vi "DC(P+V)control_KNRm.vi"(8 "control":T2, 9 "Ocmd":dbl, 10 "Tcmd":dbl, 11 "Move":T1) -> (0 "hldU":dbl, 1 "hldVerr":dbl, 2 "dirU":dbl, 3 "dirVerr":dbl, 4 "e":dbl, 5 "FriectH":dbl, 6 "dirPerr":dbl, 7 "FriectD":dbl)   [LabVIEW 2013]
uses:
  Global_KNRm.vi
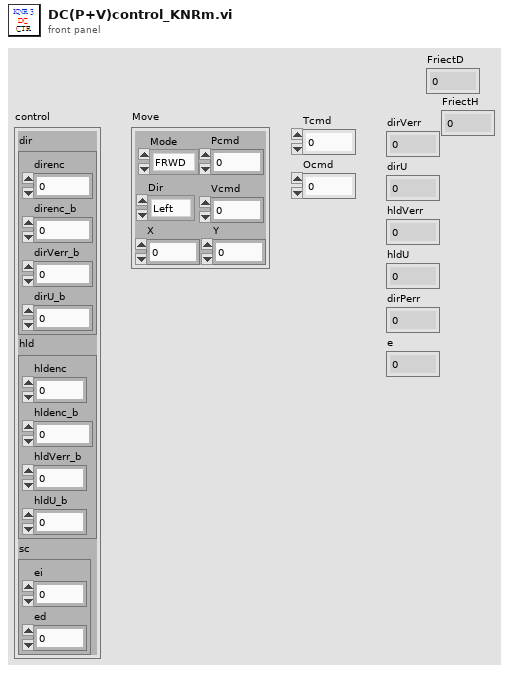
[diagram p1: front panel]
types:
  T1 = cluster{"Mode":enum16{"FRWD", "TURFIX", "TURNOF", "CIRCULAR"}, "Dir":enum16{"Left", "Right"}, "Pcmd":dbl, "Vcmd":dbl, "X":dbl, "Y":dbl}
  T2 = cluster{"dir":cluster{"direnc":dbl, "direnc_b":dbl, "dirVerr_b":dbl, "dirU_b":dbl}, "hld":cluster{"hldenc":dbl, "hldenc_b":dbl, "hldVerr_b":dbl, "hldU_b":dbl}, "sc":cluster{"ei":dbl, "ed":dbl}}
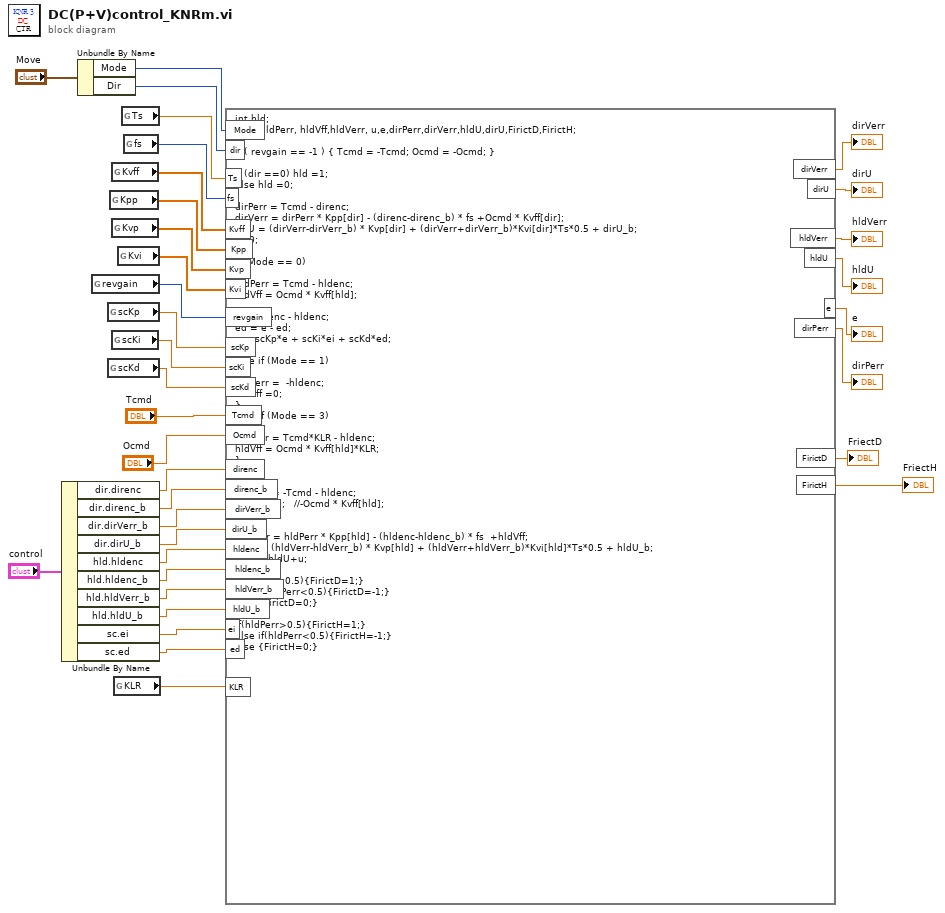
[diagram p0: block diagram]
diagram:
  n1 = Unbundle By Name("control") -> ("dir.direnc"=w19:dbl, "dir.direnc_b"=w18:dbl, "dir.dirVerr_b"=w17:dbl, "dir.dirU_b"=w16:dbl, "hld.hldenc"=w15:dbl, "hld.hldenc_b"=w14:dbl, "hld.hldVerr_b"=w13:dbl, "hld.hldU_b"=w12:dbl, "sc.ei"=w11:dbl, "sc.ed"=w10:dbl)
  n2 = Unbundle By Name("Move") -> ("Mode"=w33:enum16{"FRWD", "TURFIX", "TURNOF", "CIRCULAR"}, "Dir"=w32:enum16{"Left", "Right"})
  n3 = global read "Global_KNRm.vi" "revgain"() -> (w23:i32)
  n4 = global read "Global_KNRm.vi" "scKp"() -> (w22:dbl)
  n5 = global read "Global_KNRm.vi" "scKd"() -> (w20:dbl)
  n6 = global read "Global_KNRm.vi" "Kpp"() -> (w27:dbl[])
  n7 = global read "Global_KNRm.vi" "Kvff"() -> (w29:dbl[])
  n8 = global read "Global_KNRm.vi" "Kvp"() -> (w25:dbl[])
  n9 = global read "Global_KNRm.vi" "scKi"() -> (w21:dbl)
  n10 = global read "Global_KNRm.vi" "KLR"() -> (w1:dbl)
  n11 = global read "Global_KNRm.vi" "Kvi"() -> (w24:dbl[])
  n12 = global read "Global_KNRm.vi" "Ts"() -> (w28:dbl)
  n13 = global read "Global_KNRm.vi" "fs"() -> (w26:i32)
  n14 = formula code="int hld;\nfloat hldPerr, hldVff,hldVerr, u,e,dirPerr,dirVerr,hldU,dirU,FirictD,FirictH;\n\nif ( revgain == -1 ) { Tcmd = -Tcmd; Ocmd = -Ocmd; }\n\nif (dir ==0) hld =1;\nelse hld =0;\n\ndirPerr = Tcmd - direnc;\ndirVerr = dirPerr * Kpp[dir] - (direnc-direnc_b) * fs +Ocmd * Kvff[dir];\ndirU = (dirVerr-dirVerr_b) * Kvp[dir] + (dirVerr+dirVerr_b)*Kvi[dir]*Ts*0.5 + dirU_b;\nu=0;\n\nif (Mode == 0)\n{\nhldPerr = Tcmd - hldenc;\nhldVff = Ocmd * Kvff[hld];\n\ne = direnc - hldenc;\ned = e - ed;\nu = scKp*e + scKi*ei + scKd*ed;\n}\nelse if (Mode == 1)\n{\nhldPerr =  -hldenc;\nhldVff =0;\n}\nelse if (Mode == 3)\n{\nhldPerr = Tcmd*KLR - hldenc;\nhldVff = Ocmd * Kvff[hld]*KLR;\n}\nelse\n{\nhldPerr = -Tcmd - hldenc;\nhldVff = 0;   //-Ocmd * Kvff[hld];\n}\n\nhldVerr = hldPerr * Kpp[hld] - (hldenc-hldenc_b) * fs  +hldVff;\nhldU = (hldVerr-hldVerr_b) * Kvp[hld] + (hldVerr+hldVerr_b)*Kvi[hld]*Ts*0.5 + hldU_b;\nhldU =hldU+u;\n\nif(dirPerr>0.5){FirictD=1;}\nelse if(dirPerr<0.5){FirictD=-1;}\nelse {FirictD=0;}\n\nif(hldPerr>0.5){FirictH=1;}\nelse if(hldPerr<0.5){FirictH=-1;}\nelse {FirictH=0;}"("Mode"=w33, "dir"=w32, "Kvff"=w29, "Kpp"=w27, "Kvp"=w25, "Kvi"=w24, "revgain"=w23, "scKp"=w22, "scKi"=w21, "scKd"=w20, "Tcmd"="Tcmd", "Ocmd"="Ocmd", "Ts"=w28, "fs"=w26, "direnc"=w19, "direnc_b"=w18, "dirVerr_b"=w17, "dirU_b"=w16, "hldenc"=w15, "hldenc_b"=w14, "hldVerr_b"=w13, "hldU_b"=w12, "ei"=w11, "ed"=w10, "KLR"=w1) -> ("dirVerr"=→"dirVerr":dbl, "dirU"=→"dirU":dbl, "hldVerr"=→"hldVerr":dbl, "hldU"=→"hldU":dbl, "e"=→"e":dbl, "dirPerr"=→"dirPerr":dbl, "FirictD"=→"FriectD":dbl, "FirictH"=→"FriectH":dbl)
